vi "LED_Open.vi"(3 "error in (no error)":errorcluster) -> (7 "LED Notifier":refnum<notifier>, 10 "error out":errorcluster)   [LabVIEW 2010, in "lib1299.lvlib"]
doc: "This VI initializes the LED Loop noitifier\n\nInputs:\nerror in - error input cluster\n\nOutputs:\nLED Notifier - notifier for LED loop\nerror out - error output cluster"
uses:
  lib1299.lvlib
  TYP_LEDSegNotifier.ctl
  TYP_LEDCommand.ctl
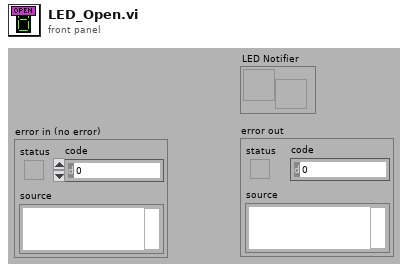
[diagram p1: front panel]
types:
  T1 = typedef "lib1299.lvlib/TYP_LEDSegNotifier.ctl" = cluster{"notification":T2, "Data":i32}
  T2 = typedef "lib1299.lvlib/TYP_LEDCommand.ctl" = enum16{"Init", "Go ACQ", "Go XFR", "Manual", "Stop", "Exit"}
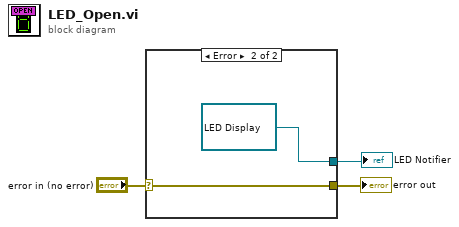
[diagram p0: block diagram]
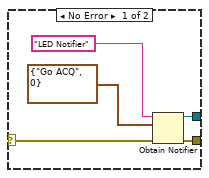
[diagram p2: hidden frame]
diagram:
  n1 = case shown="Error" "error in (no error)" {
    selector: "error in (no error)" -> [w7 w10]
    tunnel: [w8 w10] -> w3
    tunnel: [w4 refnum<notifier> refnum ("notifier out")] -> w1
    frame No Error {
      n2 = Obtain Notifier(name (unnamed)="LED Notifier", notification data type=T1 {"notification"=enum."Go ACQ", "Data"=0} ("LED Display"), error in (no error)=w7) -> (notifier out=w4:refnum<notifier>, error out=w8:errorcluster)  [unwired: 1 in, 1 out]
    }
    frame Error {
    }
  }
  "LED Notifier" <- w1
  "error out" <- w3
